vi "UATrustClientCerts.vi"(8 "error in (no error)":errorcluster, 10 "OPC UA server refnum in":refnum<k21>, 11 "Server config info":T1) -> (0 "error out":errorcluster, 1 "Array":path[](array[path]), 2 "OPC UA server refnum out":refnum<k21>, 3 "Server config info (dup)":T1)   [LabVIEW 2014, in "OPCUA XML(dev).lvlib"]
uses:
  OPCUA XML(dev).lvlib
  DEF-Server Config Data.ctl
  <vilib>/OPCUA/NI OPC UA Server.lvlib
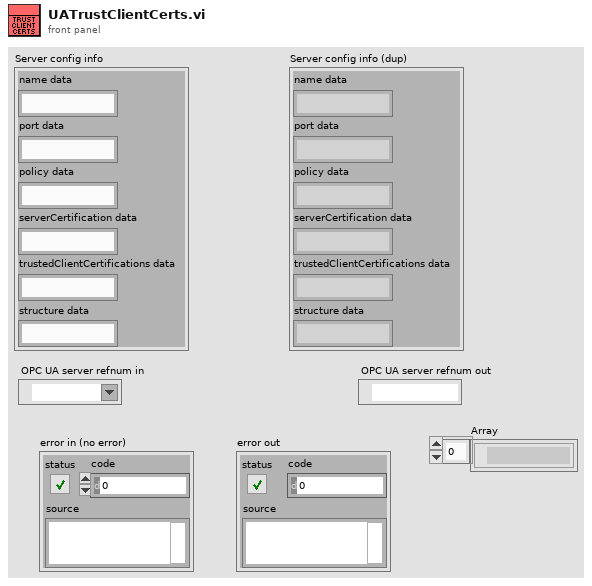
[diagram p1: front panel]
types:
  T1 = typedef "OPCUA XML(dev).lvlib/DEF-Server Config Data.ctl" = cluster{"name data":string, "port data":string, "policy data":string, "serverCertification data":string, "trustedClientCertifications data":string, "structure data":string}
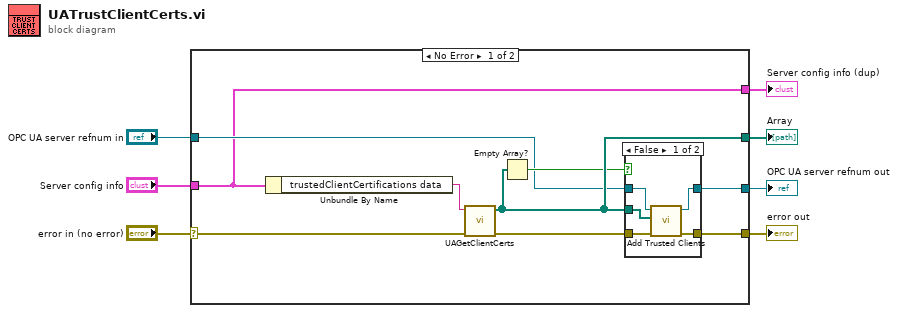
[diagram p0: block diagram]
diagram:
  n1 = case shown="No Error" "error in (no error)" {
    selector: "error in (no error)" -> [w9 w26]
    tunnel: [w16 _] -> w7
    tunnel: [w14 w26] -> w6
    tunnel: "Server config info" -> [w8 w24]
    tunnel: "OPC UA server refnum in" -> [w11 w25]
    tunnel: [w10 w25] -> w3
    tunnel: [w8 w24] -> w1
    frame No Error {
      n2 = Unbundle By Name(w8) -> ("trustedClientCertifications data"=w12:string)
      n3 = call "UAGetClientCerts.vi"("error in (no error)"=w9, "trustedClientCertifications data"=w12) -> ("error out"=w13:errorcluster, "Array"=w16:path[])  [unwired: 8 in]
      n4 = Empty Array?(array=w16) -> (empty?=w15:bool)
      n5 = case shown="False" w15 {
        tunnel: w13 -> [w21 w23]
        tunnel: [w20 w23] -> w14
        tunnel: w16 -> [w19 _]
        tunnel: w11 -> [w18 w22]
        tunnel: [w17 w22] -> w10
        frame False {
          n6 = call <vilib>:"Add Trusted Clients.vi"("error in (no error)"=w21, "trusted client certificates"=w19, "OPC UA server refnum in"=w18) -> ("error out"=w20:errorcluster, "OPC UA server refnum out"=w17:refnum<k21>)  [unwired: 7 in]
        }
        frame True {
        }
      }
    }
    frame Error {
    }
  }
  "Array" <- w7
  "error out" <- w6
  "Server config info (dup)" <- w1
  "OPC UA server refnum out" <- w3
